vi "SaveLockinSweepData.vi"(8 "error in (no error)":errorcluster, 9 "Sweep_AI":waveform(dbl)[](array[waveform]), 10 "Sweep_AO":waveform(dbl)[](array[waveform]), 11 "AFM_Litho_Plugin.IV in":refnum<class "AFM_Litho_Plugin.IV.lvclass">) -> (0 "error out":errorcluster, 3 "AFM_Litho_Plugin.IV out":refnum<class "AFM_Litho_Plugin.IV.lvclass">)   [LabVIEW 2019, in "AFM_Litho_Plugin.IV.lvclass"]
uses:
  AFM_Litho_Plugin.IV.lvclass
  <userlib>/LevyLab/LV-Data/LV-Data/Typedefs/File Type--enum.ctl
  AFM_Litho_Plugin.IV.lvclass/AFM_Litho_Plugin.IV.ctl
  <userlib>/LevyLab/LV-Data/LV-Data/Typedefs/Dictionary--cluster.ctl
  <userlib>/LevyLab/LV-Data/LV-Data/LV-Data.lvclass
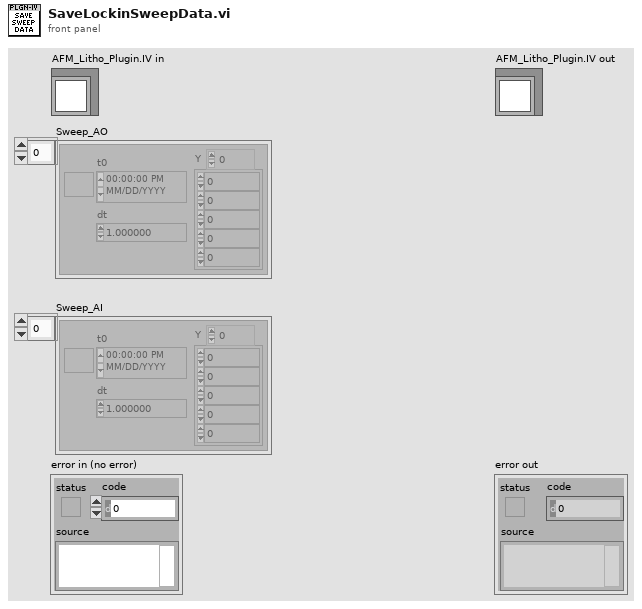
[diagram p1: front panel]
types:
  T1 = typedef "LV-Data.lvclass/File Type--enum.ctl" = enum16{"DAT", "ITX", "TDMS", "VI"}
  T2 = typedef "LV-Data.lvclass/Dictionary--cluster.ctl" = cluster{"key":string, "value":variant}
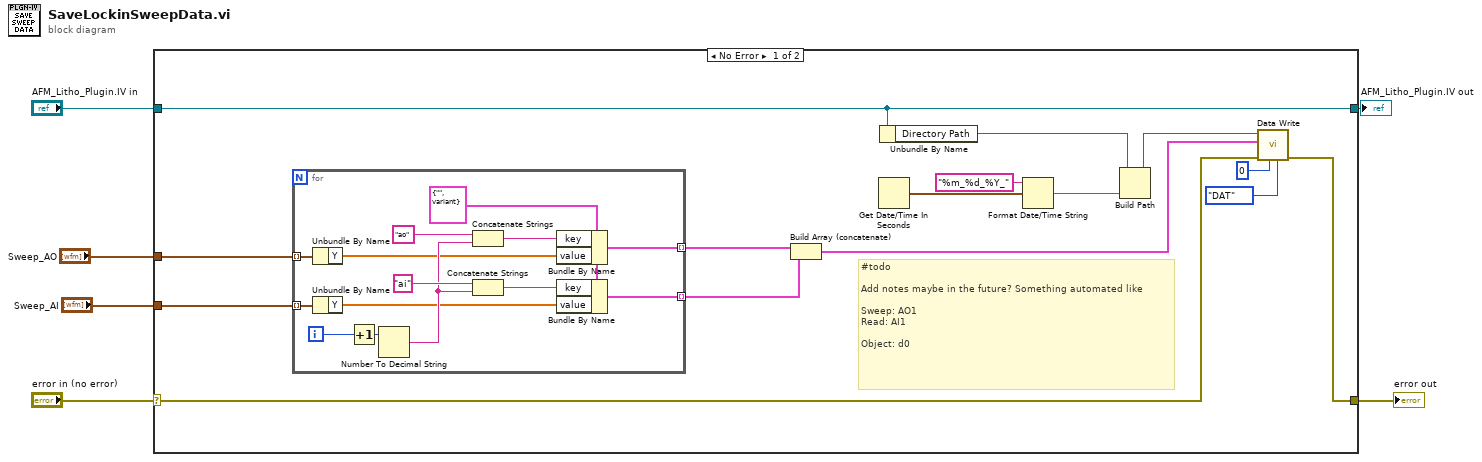
[diagram p0: block diagram]
diagram:
  n1 = case shown="No Error" "error in (no error)" {
    selector: "error in (no error)" -> [w11 w37]
    tunnel: [w10 w37] -> w5
    tunnel: [w21 w36] -> w3
    tunnel: "AFM_Litho_Plugin.IV in" -> [w21 w36]
    tunnel: "Sweep_AI" -> [w16 _]
    tunnel: "Sweep_AO" -> [w15 _]
    frame No Error {
      # "#todo\n\nAdd notes maybe in the future? Something automated like \n\nSweep: AO1\nRead: AI1\n\nObject: d0"
      n2 = for {
        tunnel: w15 -> [w29] mode=indexing
        tunnel: w16 -> [w27] mode=indexing
        tunnel: [w25] -> w17 mode=indexing
        tunnel: [w23] -> w14 mode=indexing
        i -> [w35]
        w24 = T2 {"key"="", "value"=variant} ("key-value")
        n3 = Unbundle By Name(w29) -> ("Y"=w28:dbl[])
        n4 = Unbundle By Name(w27) -> ("Y"=w26:dbl[])
        n5 = Increment(x=w35) -> (x+1=w22:i32)
        n6 = Number To Decimal String(number=w22) -> (decimal integer string=w32:string)  [unwired: 1 in]
        n7 = Concatenate Strings("ao", w32) -> (w30:string)
        n8 = Concatenate Strings("ai", w32) -> (w31:string)
        n9 = Bundle By Name(cluster=w24, "key"=w30, "value"=w28) -> (w23:T2)
        n10 = Bundle By Name(cluster=w24, "key"=w31, "value"=w26) -> (w25:T2)
      }
      n11 = Build Array (concatenate)(w14, w17) -> (w7:T2[])
      n12 = Get Date/Time In Seconds() -> (seconds since 1Jan1904=w19:timestamp)
      n13 = Unbundle By Name(w21) -> ("Directory Path"=w9:path)
      n14 = Format Date/Time String(time format string (%c)="%m_%d_%Y_", seconds (now)=w19) -> (date/time string=w18:string)  [unwired: 1 in]
      n15 = Build Path(base path=w9, name or relative path=w18) -> (appended path=w8:path)
      n16 = call <userlib>:"Data Write.vi"("File Type"=File_Type--enum."DAT", "Append Index"=0, "error in (no error)"=w11, "Data (Dictionary)"=w7, "path"=w8) -> ("error out"=w10:errorcluster)  [unwired: 5 in, 1 out]
    }
    frame Error {
    }
  }
  "error out" <- w5
  "AFM_Litho_Plugin.IV out" <- w3
